vi "Shifter.vi"(3 "Shift":bool) -> ()   [LabVIEW 2017]
uses:
  <vilib>/Rock Robotics/WPI/Solenoid/Deprecated/WPI_SolenoidSetBool.vi
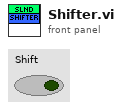
[diagram p1: front panel]
types:
  T1 = typedef "WPI_SolenoidDevRef.ctl" = cluster{"DevStatus":errorcluster, "Pneumatics Control Module":u8, "Forward Solenoid Channel":T2, "Reverse Solenoid Channel":T2}
  T2 = typedef "WPI_SolenoidChannel.ctl" = enum8{"Solenoid 0", "Solenoid 1", "Solenoid 2", "Solenoid 3", "Solenoid 4", "Solenoid 5", "Solenoid 6", "Solenoid 7", "Invalid"}
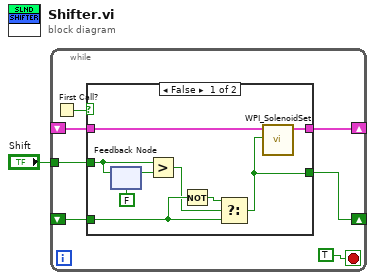
[diagram p0: block diagram]
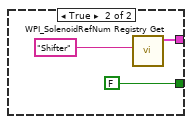
[diagram p2: hidden frame]
diagram:
  n1 = while {
    shift-right: [w5] -> _
    shift-left: _ -> [w6]
    shift-right: [w4] -> _
    shift-left: _ -> [w3]
    tunnel: "Shift" -> [w2]
    stop <- TRUE stop-if-true
    n2 = First Call?() -> (First Call?: T/F=w7:bool)
    n3 = case shown="False" w7 {
      tunnel: w6 -> [w13 _]
      tunnel: [w15 FALSE ("Shift")] -> w5
      tunnel: [w16 w19] -> w4
      tunnel: w3 -> [w17 _]
      tunnel: w2 -> [w10 _]
      frame False {
        n4 = feedback #1(FALSE) -> (w12:bool)
        n5 = feedback-in #1(w10) -> ()
        n6 = Greater?(x=w10, y=w12) -> (0:w9:bool)
        n7 = Not(x=w13) -> (.not. x?=w14:bool)
        n8 = Select(t=w14, s=w9, f=w13) -> (s? t:f=w15:bool)
        n9 = call-poly <vilib>:"WPI_SolenoidSet.vi"("Value"=w15, "SolenoidDevRef"=w17) -> ("SolenoidDevRef"=w16:T1)  [unwired: 8 in, 1 out]
      }
      frame True {
        n10 = call <vilib>:"WPI_SolenoidRefNum Registry Get.vi"("refnum name"="Shifter") -> ("SolenoidDevRef"=w19:T1)  [unwired: 9 in, 1 out]
      }
    }
  }
